vi "CALL_NI.vi"(10 "banco":i32, 11 "simulazione":bool) -> ()   [LabVIEW 2019]
panel:
  out "Loop Iteration":i32
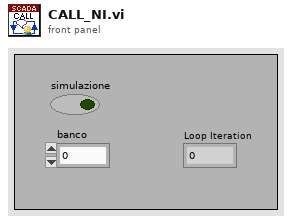
[diagram p1: front panel]
types:
  T1 = enum16{"Left Button", "Center Button", "Right Button", "Window Close"}
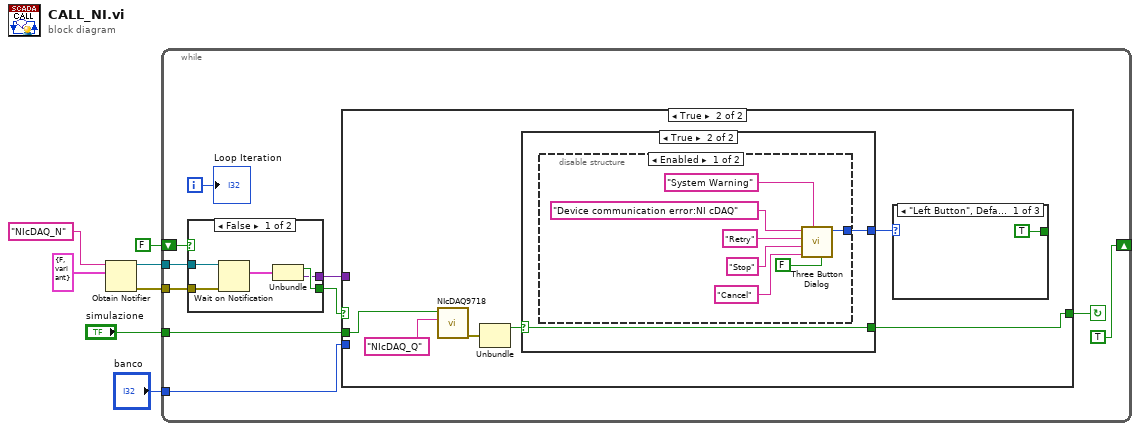
[diagram p0: block diagram]
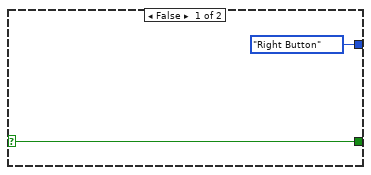
[diagram p4: hidden frame]
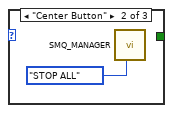
[diagram p6: hidden frame]
diagram:
  n1 = Obtain Notifier(name (unnamed)="NIcDAQ_N" ("Notifier Name"), notification data type=cluster{"boolean":bool, "variant":variant} {"boolean"=FALSE, "variant"=variant} ("notification")) -> (notifier out=w5:refnum<notifier>, error out=w6:errorcluster)  [unwired: 2 in, 1 out]
  n2 = while {
    tunnel: "simulazione" -> [w16]
    tunnel: w6 -> [w14]
    tunnel: w5 -> [w15]
    shift-right: [TRUE] -> _
    shift-left: FALSE -> [w11]
    tunnel: "banco" -> [w9]
    i -> [w8]
    stop <- w17 continue-if-true
    n3 = case shown="False" w11 {
      selector: w11 -> [_ w23]
      tunnel: w15 -> [w22 _]
      tunnel: w14 -> [w21 _]
      tunnel: [w19 w23] -> w13
      tunnel: [w18 _] -> w12
      frame False {
        n4 = Wait on Notification(notifier=w22, error in (no error)=w21) -> (notification=w20:cluster{"boolean":bool, "variant":variant})  [unwired: 2 in, 3 out]
        n5 = Unbundle(w20) -> ("boolean"=w19:bool, "variant"=w18:variant)
      }
      frame True {
      }
    }
    n6 = case shown="True" w13 {
      selector: w13 -> [w24 _]
      tunnel: [w24 w26] -> w17
      tunnel: w12 -> [_ _]
      tunnel: w16 -> [_ w25]
      tunnel: w9 -> [_ _]
      frame False {
      }
      frame True {
        n7 = call "NIcDAQ9718.vi"("Queue Name"="NIcDAQ_Q", "Simulation"=w25) -> ("error out"=w27:errorcluster)  [unwired: 9 in]
        n8 = Unbundle(w27) -> ("status"=w30:bool)  [unwired: 2 out]
        n9 = case shown="True" w30 {
          selector: w30 -> [w31 w33]
          tunnel: [T1."Right Button" ("Which Button?") w34] -> w29
          tunnel: [w31 w33] -> w26
          frame False {
          }
          frame True {
            n10 = disable-structure shown="Enabled" {
              disable-tunnel: [w35 _] -> w34
              frame Enabled {
                n11 = call <vilib>:"Three Button Dialog.vi"("Allow user to close window? (TRUE)"=FALSE, "Window Title (\"\")"="System Warning" ("Window Title (\"\")"), "Right Button Text (\"Cancel\")"="Cancel" ("Right Button Text (\"Cancel\")"), "Center Button Text (\"No\")"="Stop" ("Center Button Text (\"No\")"), "Left Button Text (\"Yes\")"="Retry" ("Left Button Text (\"Yes\")"), "message"="Device communication error:NI cDAQ") -> ("Which Button?"=w35:T1)  [unwired: 5 in]
              }
              frame Disabled {
              }
            }
          }
        }
        n12 = case shown="\"Left Button\", Default" w29 {
          tunnel: [TRUE ("Allow user to close window? (TRUE)") _ _] -> _
          frame "Left Button", Default {
          }
          frame "Center Button" {
            n13 = call <userlib>:"SMQ_MANAGER.vi"("Function"=enum16{"INITIALIZE", "ENQUEUE", "STOP ALL"}."STOP ALL") -> ()  [unwired: 10 in, 1 out]
          }
          frame "Right Button" {
          }
        }
      }
    }
    "Loop Iteration" <- w8
  }
